vi "get flash file path.vi"(11 "Part Type":string) -> (3 "flash file path":path)   [LabVIEW 2018]
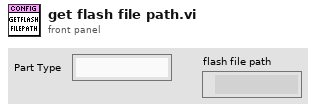
[diagram p1: front panel]
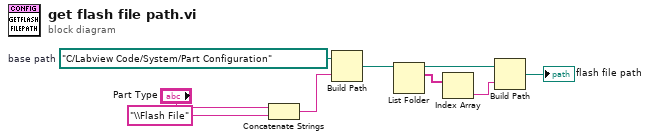
[diagram p0: block diagram]
diagram:
  w5 = path "C:/Labview Code/System/Part Configuration"  # base path
  n1 = Concatenate Strings("Part Type", "\\Flash File") -> (w2:string)
  n2 = Build Path(base path=w5, name or relative path=w2) -> (appended path=w6:path)
  n3 = List Folder(path=w6) -> (path out=w7:path, filenames=w8:string[])  [unwired: 3 in, 2 out]
  n4 = Index Array(array=w8) -> (element=w9:string)  [unwired: 1 in]
  n5 = Build Path(base path=w7, name or relative path=w9) -> (appended path=→"flash file path":path)
